vi "Task Manager.vi"() -> ()   [LabVIEW 2017]
doc: "Use this template to build a user interface event handler design pattern. Use this pattern for dialog boxes and other user interfaces. You also can create and execute user-defined events that the VI can handle the same way as user interface events."
uses:
  Task View Control.ctl
panel:
  in  "Advance":bool
  out "Input Task Tip":string
  in  "Input Value":string caption="Thermocouple Reading"
  out "Task Tip":string
  out "Experiment Progress":u8(slide) scale=0.0..15.0
  in  "?":bool
  out "tracker2":bool caption="Item 2"
  out "tracker5":bool caption="Item 5"
  out "tracker3":bool caption="Item 3"
  out "tracker1":bool caption="Item 1"
  out "tracker4":bool caption="Item 4"
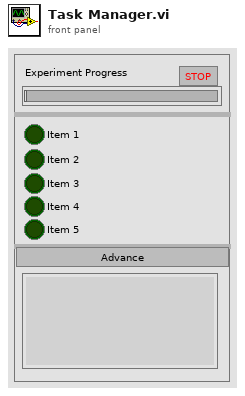
[diagram p1: front panel]
types:
  T1 = typedef "Task View Control.ctl" = enum16{"init", "Activate Pump 1", "Activate CTAH 1", "Set Pump Freq to 10Hz 1", "Vary Pump Freqs 1", "Vary Pump Freqs 2", "Stop Pump 1", "Stop Pump 2", "Ramp Up Pump Freq 1", "Ramp Up Pump Freq 2", "Ramp Up Pump Freq 3", "Ramp Up Pump Freq 4", "Ramp Up Power 1", "Ramp Up Power 2", "Ramp up Power 3", "Ramp up Power 4", "Ramp up Power 5", "Set CTAH 1", "Set CTAH 2", "Set CTAH 3", "Change Pump Freq", "Run Input 1", "Run Input 2", "Turn Off Power 1", "Turn Off Power 2", "Turn Off Power 3", "Primary Loop Cooldown 1", "Primary Loop Cooldown 2", "Primary Loop Cooldown 3", "Turn off CTAH", "Turn off chat", "complete"}
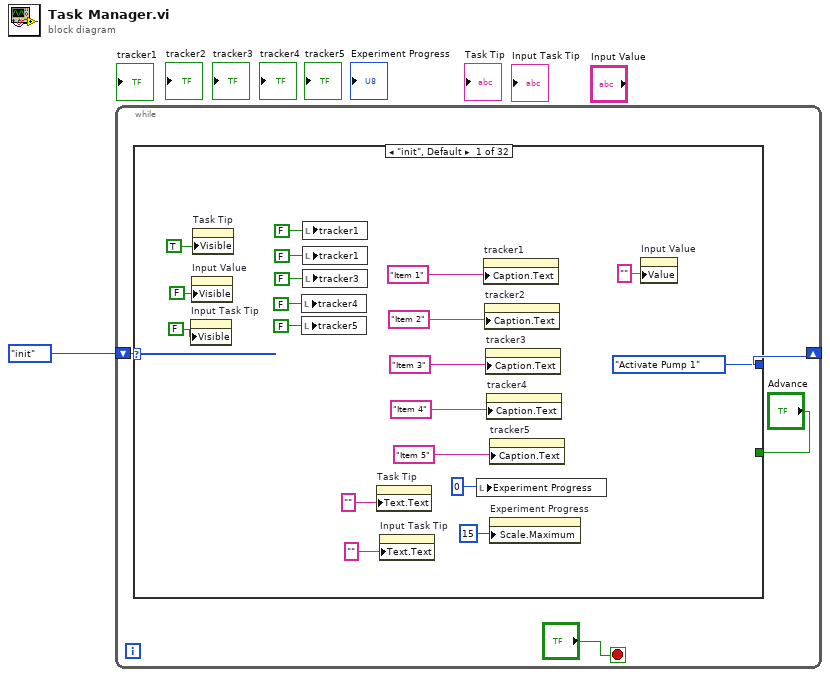
[diagram p0: block diagram]
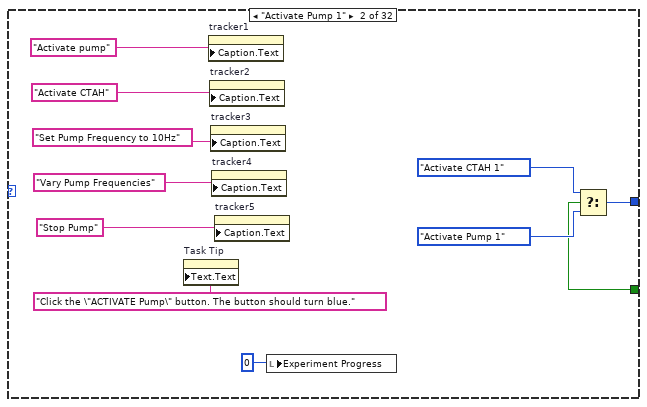
[diagram p2: hidden frame]
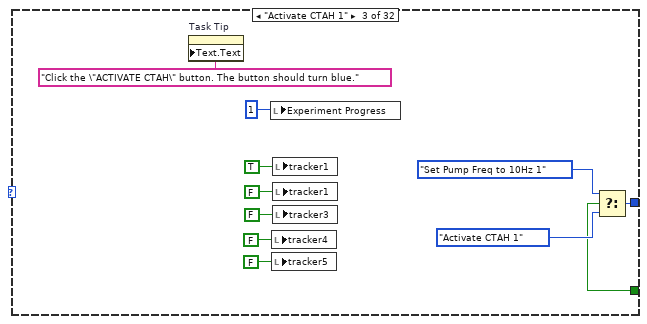
[diagram p3: hidden frame]
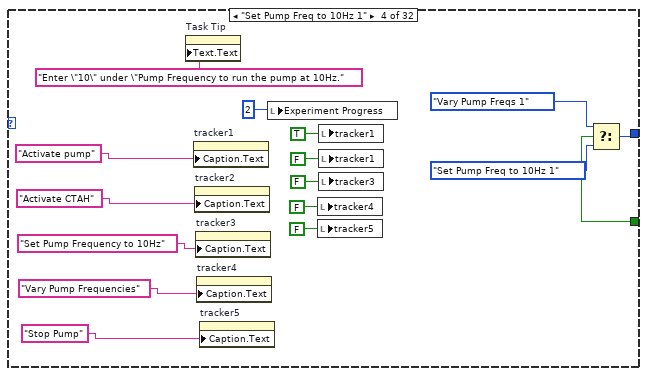
[diagram p4: hidden frame]
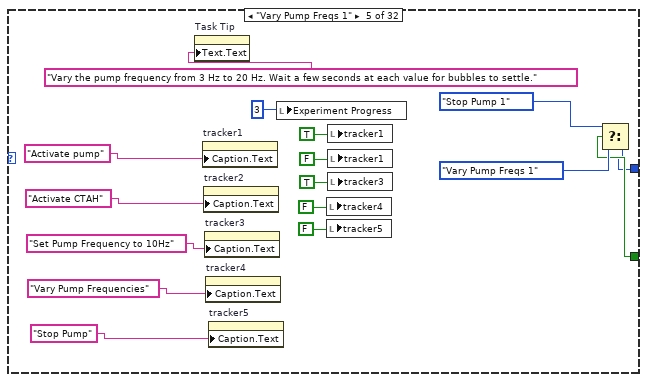
[diagram p5: hidden frame]
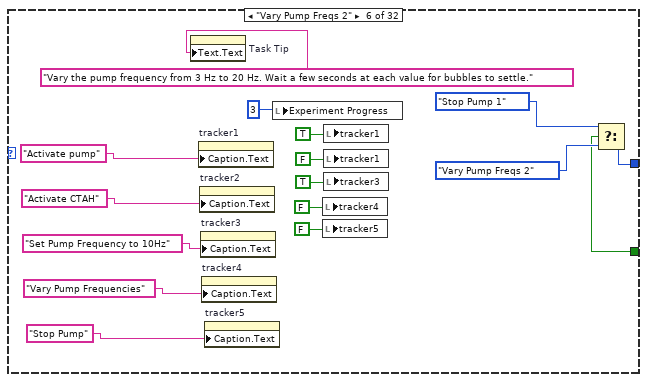
[diagram p6: hidden frame]
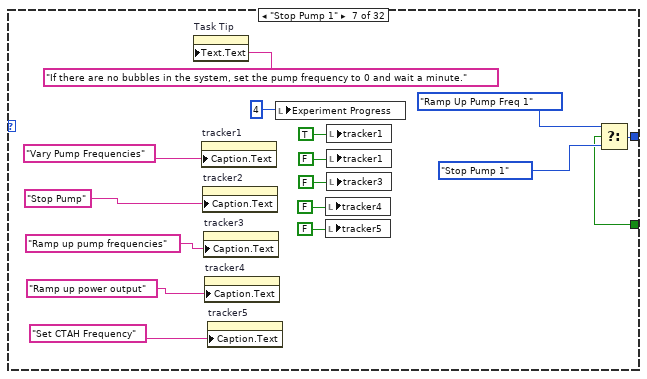
[diagram p7: hidden frame]
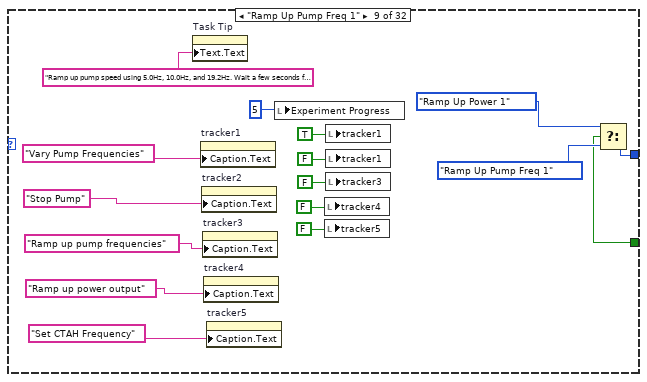
[diagram p9: hidden frame]
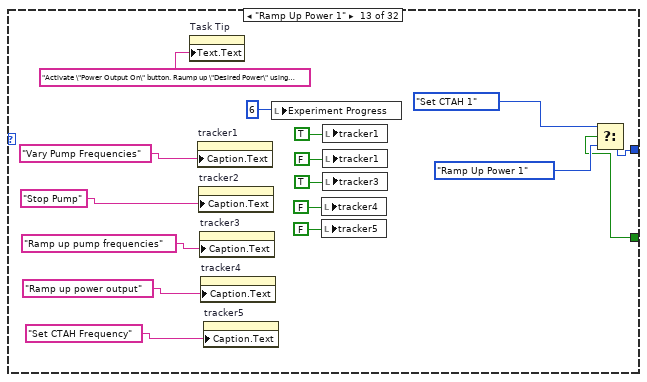
[diagram p13: hidden frame]
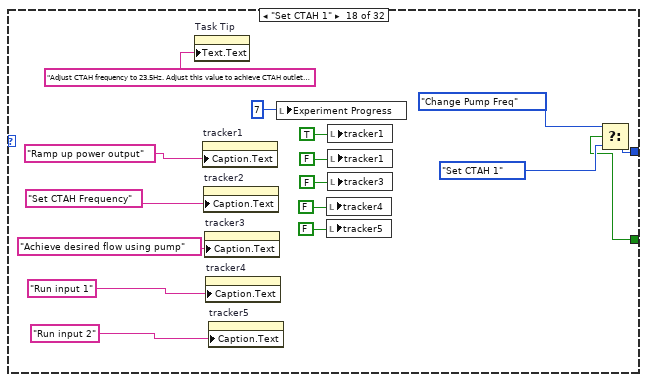
[diagram p18: hidden frame]
diagram:
  n1 = while {
    shift-right: [w3] -> _
    shift-left: Task_View_Control."init" -> [w4]
    stop <- "?" stop-if-true
    n2 = case shown="\"init\", Default" w4 {
      tunnel: [Task_View_Control."Activate Pump 1" w29 w45 w63 w66 w83 w100 _ w117 _ _ _ w134 _ _ _ _ w151 _ _ w168 w186 w202 w220 _ _ w236 _ _ w253 w270 w289] -> w3
      tunnel: "Advance" -> [_ w26 w43 w60 w67 w84 w101 _ w118 _ _ _ w135 _ _ _ _ w152 _ _ w169 w185 w203 w219 _ _ w237 _ _ w254 w271 w288]
      frame "init", Default {
        n3 = property on="Input Task Tip" class="Str"("Visible"=FALSE) -> ()  [unwired: 2 in, 2 out]
        n4 = property on="Input Value" class="Str"("Visible"=FALSE) -> ()  [unwired: 2 in, 2 out]
        n5 = property on="Task Tip" class="Str"("Visible"=TRUE) -> ()  [unwired: 2 in, 2 out]
        n6 = local write "tracker4"(FALSE) -> ()
        n7 = local write "tracker5"(FALSE) -> ()
        n8 = local write "tracker1"(FALSE) -> ()
        n9 = local write "tracker2"(FALSE) -> ()
        n10 = local write "tracker1"(FALSE) -> ()
        n11 = local write "tracker3"(FALSE) -> ()
        n12 = property on="Task Tip" class="Str"("Text.Text"="") -> ()  [unwired: 2 in, 2 out]
        n13 = property on="Input Task Tip" class="Str"("Text.Text"="") -> ()  [unwired: 2 in, 2 out]
        n14 = local write "Experiment Progress"(0) -> ()
        n15 = property on="tracker1" class="Bool (strict)"("Caption.Text"="Item 1") -> ()  [unwired: 2 in, 2 out]
        n16 = property on="tracker2" class="Bool (strict)"("Caption.Text"="Item 2") -> ()  [unwired: 2 in, 2 out]
        n17 = property on="tracker3" class="Bool (strict)"("Caption.Text"="Item 3") -> ()  [unwired: 2 in, 2 out]
        n18 = property on="tracker4" class="Bool (strict)"("Caption.Text"="Item 4") -> ()  [unwired: 2 in, 2 out]
        n19 = property on="tracker5" class="Bool (strict)"("Caption.Text"="Item 5") -> ()  [unwired: 2 in, 2 out]
        n20 = property on="Experiment Progress" class="Slide (strict)"("Scale.Maximum"=15) -> ()  [unwired: 2 in, 2 out]
        n21 = property on="Input Value" class="Str"("Value"="") -> ()  [unwired: 2 in, 2 out]
      }
      frame "Activate Pump 1" {
        n22 = property on="Task Tip" class="Str"("Text.Text"="Click the \"ACTIVATE Pump\" button. The button should turn blue.") -> ()  [unwired: 2 in, 2 out]
        n23 = property on="tracker1" class="Bool (strict)"("Caption.Text"="Activate pump") -> ()  [unwired: 2 in, 2 out]
        n24 = property on="tracker2" class="Bool (strict)"("Caption.Text"="Activate CTAH") -> ()  [unwired: 2 in, 2 out]
        n25 = property on="tracker3" class="Bool (strict)"("Caption.Text"="Set Pump Frequency to 10Hz") -> ()  [unwired: 2 in, 2 out]
        n26 = property on="tracker4" class="Bool (strict)"("Caption.Text"="Vary Pump Frequencies") -> ()  [unwired: 2 in, 2 out]
        n27 = property on="tracker5" class="Bool (strict)"("Caption.Text"="Stop Pump") -> ()  [unwired: 2 in, 2 out]
        n28 = local write "Experiment Progress"(0) -> ()
        n29 = Select(t=Task_View_Control."Activate CTAH 1", s=w26, f=Task_View_Control."Activate Pump 1") -> (s? t:f=w29:T1)
      }
      frame "Activate CTAH 1" {
        n30 = property on="Task Tip" class="Str"("Text.Text"="Click the \"ACTIVATE CTAH\" button. The button should turn blue.") -> ()  [unwired: 2 in, 2 out]
        n31 = local write "Experiment Progress"(1) -> ()
        n32 = local write "tracker4"(FALSE) -> ()
        n33 = local write "tracker5"(FALSE) -> ()
        n34 = local write "tracker1"(TRUE) -> ()
        n35 = local write "tracker2"(FALSE) -> ()
        n36 = local write "tracker1"(FALSE) -> ()
        n37 = local write "tracker3"(FALSE) -> ()
        n38 = Select(t=Task_View_Control."Set Pump Freq to 10Hz 1", s=w43, f=Task_View_Control."Activate CTAH 1") -> (s? t:f=w45:T1)
      }
      frame "Set Pump Freq to 10Hz 1" {
        n39 = property on="Task Tip" class="Str"("Text.Text"="Enter \"10\" under \"Pump Frequency to run the pump at 10Hz.") -> ()  [unwired: 2 in, 2 out]
        n40 = property on="tracker1" class="Bool (strict)"("Caption.Text"="Activate pump") -> ()  [unwired: 2 in, 2 out]
        n41 = property on="tracker2" class="Bool (strict)"("Caption.Text"="Activate CTAH") -> ()  [unwired: 2 in, 2 out]
        n42 = property on="tracker3" class="Bool (strict)"("Caption.Text"="Set Pump Frequency to 10Hz") -> ()  [unwired: 2 in, 2 out]
        n43 = property on="tracker4" class="Bool (strict)"("Caption.Text"="Vary Pump Frequencies") -> ()  [unwired: 2 in, 2 out]
        n44 = property on="tracker5" class="Bool (strict)"("Caption.Text"="Stop Pump") -> ()  [unwired: 2 in, 2 out]
        n45 = local write "Experiment Progress"(2) -> ()
        n46 = local write "tracker4"(FALSE) -> ()
        n47 = local write "tracker5"(FALSE) -> ()
        n48 = local write "tracker1"(TRUE) -> ()
        n49 = local write "tracker2"(TRUE) -> ()
        n50 = local write "tracker1"(FALSE) -> ()
        n51 = local write "tracker3"(FALSE) -> ()
        n52 = Select(t=Task_View_Control."Vary Pump Freqs 1", s=w60, f=Task_View_Control."Set Pump Freq to 10Hz 1") -> (s? t:f=w63:T1)
      }
      frame "Vary Pump Freqs 1" {
        n53 = property on="Task Tip" class="Str"("Text.Text"="Vary the pump frequency from 3 Hz to 20 Hz. Wait a few seconds at each value for bubbles to settle.") -> ()  [unwired: 2 in, 2 out]
        n54 = property on="tracker1" class="Bool (strict)"("Caption.Text"="Activate pump") -> ()  [unwired: 2 in, 2 out]
        n55 = property on="tracker2" class="Bool (strict)"("Caption.Text"="Activate CTAH") -> ()  [unwired: 2 in, 2 out]
        n56 = property on="tracker3" class="Bool (strict)"("Caption.Text"="Set Pump Frequency to 10Hz") -> ()  [unwired: 2 in, 2 out]
        n57 = property on="tracker4" class="Bool (strict)"("Caption.Text"="Vary Pump Frequencies") -> ()  [unwired: 2 in, 2 out]
        n58 = property on="tracker5" class="Bool (strict)"("Caption.Text"="Stop Pump") -> ()  [unwired: 2 in, 2 out]
        n59 = local write "Experiment Progress"(3) -> ()
        n60 = local write "tracker4"(FALSE) -> ()
        n61 = local write "tracker5"(FALSE) -> ()
        n62 = local write "tracker1"(TRUE) -> ()
        n63 = local write "tracker2"(TRUE) -> ()
        n64 = local write "tracker1"(FALSE) -> ()
        n65 = local write "tracker3"(TRUE) -> ()
        n66 = Select(t=Task_View_Control."Stop Pump 1", s=w67, f=Task_View_Control."Vary Pump Freqs 1") -> (s? t:f=w66:T1)
      }
      frame "Vary Pump Freqs 2" {
        n67 = property on="Task Tip" class="Str"("Text.Text"="Vary the pump frequency from 3 Hz to 20 Hz. Wait a few seconds at each value for bubbles to settle.") -> ()  [unwired: 2 in, 2 out]
        n68 = property on="tracker1" class="Bool (strict)"("Caption.Text"="Activate pump") -> ()  [unwired: 2 in, 2 out]
        n69 = property on="tracker2" class="Bool (strict)"("Caption.Text"="Activate CTAH") -> ()  [unwired: 2 in, 2 out]
        n70 = property on="tracker3" class="Bool (strict)"("Caption.Text"="Set Pump Frequency to 10Hz") -> ()  [unwired: 2 in, 2 out]
        n71 = property on="tracker4" class="Bool (strict)"("Caption.Text"="Vary Pump Frequencies") -> ()  [unwired: 2 in, 2 out]
        n72 = property on="tracker5" class="Bool (strict)"("Caption.Text"="Stop Pump") -> ()  [unwired: 2 in, 2 out]
        n73 = local write "Experiment Progress"(3) -> ()
        n74 = local write "tracker4"(FALSE) -> ()
        n75 = local write "tracker5"(FALSE) -> ()
        n76 = local write "tracker1"(TRUE) -> ()
        n77 = local write "tracker2"(TRUE) -> ()
        n78 = local write "tracker1"(FALSE) -> ()
        n79 = local write "tracker3"(TRUE) -> ()
        n80 = Select(t=Task_View_Control."Stop Pump 1", s=w84, f=Task_View_Control."Vary Pump Freqs 2") -> (s? t:f=w83:T1)
      }
      frame "Stop Pump 1" {
        n81 = property on="Task Tip" class="Str"("Text.Text"="If there are no bubbles in the system, set the pump frequency to 0 and wait a minute.") -> ()  [unwired: 2 in, 2 out]
        n82 = property on="tracker1" class="Bool (strict)"("Caption.Text"="Vary Pump Frequencies") -> ()  [unwired: 2 in, 2 out]
        n83 = property on="tracker2" class="Bool (strict)"("Caption.Text"="Stop Pump") -> ()  [unwired: 2 in, 2 out]
        n84 = property on="tracker3" class="Bool (strict)"("Caption.Text"="Ramp up pump frequencies") -> ()  [unwired: 2 in, 2 out]
        n85 = property on="tracker4" class="Bool (strict)"("Caption.Text"="Ramp up power output") -> ()  [unwired: 2 in, 2 out]
        n86 = property on="tracker5" class="Bool (strict)"("Caption.Text"="Set CTAH Frequency") -> ()  [unwired: 2 in, 2 out]
        n87 = local write "Experiment Progress"(4) -> ()
        n88 = local write "tracker4"(FALSE) -> ()
        n89 = local write "tracker5"(FALSE) -> ()
        n90 = local write "tracker1"(TRUE) -> ()
        n91 = local write "tracker2"(FALSE) -> ()
        n92 = local write "tracker1"(FALSE) -> ()
        n93 = local write "tracker3"(FALSE) -> ()
        n94 = Select(t=Task_View_Control."Ramp Up Pump Freq 1", s=w101, f=Task_View_Control."Stop Pump 1") -> (s? t:f=w100:T1)
      }
      frame "Stop Pump 2" {
      }
      frame "Ramp Up Pump Freq 1" {
        n95 = property on="Task Tip" class="Str"("Text.Text"="Ramp up pump speed using 5.0Hz, 10.0Hz, and 19.2Hz. Wait a few seconds for the system to settle at each value. Change the final value to achieve a mass flow of 0.18 kg/s.") -> ()  [unwired: 2 in, 2 out]
        n96 = property on="tracker1" class="Bool (strict)"("Caption.Text"="Vary Pump Frequencies") -> ()  [unwired: 2 in, 2 out]
        n97 = property on="tracker2" class="Bool (strict)"("Caption.Text"="Stop Pump") -> ()  [unwired: 2 in, 2 out]
        n98 = property on="tracker3" class="Bool (strict)"("Caption.Text"="Ramp up pump frequencies") -> ()  [unwired: 2 in, 2 out]
        n99 = property on="tracker4" class="Bool (strict)"("Caption.Text"="Ramp up power output") -> ()  [unwired: 2 in, 2 out]
        n100 = property on="tracker5" class="Bool (strict)"("Caption.Text"="Set CTAH Frequency") -> ()  [unwired: 2 in, 2 out]
        n101 = local write "Experiment Progress"(5) -> ()
        n102 = local write "tracker4"(FALSE) -> ()
        n103 = local write "tracker5"(FALSE) -> ()
        n104 = local write "tracker1"(TRUE) -> ()
        n105 = local write "tracker2"(TRUE) -> ()
        n106 = local write "tracker1"(FALSE) -> ()
        n107 = local write "tracker3"(FALSE) -> ()
        n108 = Select(t=Task_View_Control."Ramp Up Power 1", s=w118, f=Task_View_Control."Ramp Up Pump Freq 1") -> (s? t:f=w117:T1)
      }
      frame "Ramp Up Pump Freq 2" {
      }
      frame "Ramp Up Pump Freq 3" {
      }
      frame "Ramp Up Pump Freq 4" {
      }
      frame "Ramp Up Power 1" {
        n109 = property on="Task Tip" class="Str"("Text.Text"="Activate \"Power Output On\" button. Raump up \"Desired Power\" using 500W, 2000W, 4000W, 6000W, 8000W. Wait for 10 seconds at each value.") -> ()  [unwired: 2 in, 2 out]
        n110 = property on="tracker1" class="Bool (strict)"("Caption.Text"="Vary Pump Frequencies") -> ()  [unwired: 2 in, 2 out]
        n111 = property on="tracker2" class="Bool (strict)"("Caption.Text"="Stop Pump") -> ()  [unwired: 2 in, 2 out]
        n112 = property on="tracker3" class="Bool (strict)"("Caption.Text"="Ramp up pump frequencies") -> ()  [unwired: 2 in, 2 out]
        n113 = property on="tracker4" class="Bool (strict)"("Caption.Text"="Ramp up power output") -> ()  [unwired: 2 in, 2 out]
        n114 = property on="tracker5" class="Bool (strict)"("Caption.Text"="Set CTAH Frequency") -> ()  [unwired: 2 in, 2 out]
        n115 = local write "Experiment Progress"(6) -> ()
        n116 = local write "tracker4"(FALSE) -> ()
        n117 = local write "tracker5"(FALSE) -> ()
        n118 = local write "tracker1"(TRUE) -> ()
        n119 = local write "tracker2"(TRUE) -> ()
        n120 = local write "tracker1"(FALSE) -> ()
        n121 = local write "tracker3"(TRUE) -> ()
        n122 = Select(t=Task_View_Control."Set CTAH 1", s=w135, f=Task_View_Control."Ramp Up Power 1") -> (s? t:f=w134:T1)
      }
      frame "Ramp Up Power 2" {
      }
      frame "Ramp up Power 3" {
      }
      frame "Ramp up Power 4" {
      }
      frame "Ramp up Power 5" {
      }
      frame "Set CTAH 1" {
        n123 = property on="Task Tip" class="Str"("Text.Text"="Adjust CTAH frequency to 23.5Hz. Adjust this value to achieve CTAH outlet temperature of 80°C.") -> ()  [unwired: 2 in, 2 out]
        n124 = property on="tracker1" class="Bool (strict)"("Caption.Text"="Ramp up power output") -> ()  [unwired: 2 in, 2 out]
        n125 = property on="tracker2" class="Bool (strict)"("Caption.Text"="Set CTAH Frequency") -> ()  [unwired: 2 in, 2 out]
        n126 = property on="tracker3" class="Bool (strict)"("Caption.Text"="Achieve desired flow using pump") -> ()  [unwired: 2 in, 2 out]
        n127 = property on="tracker4" class="Bool (strict)"("Caption.Text"="Run input 1") -> ()  [unwired: 2 in, 2 out]
        n128 = property on="tracker5" class="Bool (strict)"("Caption.Text"="Run input 2") -> ()  [unwired: 2 in, 2 out]
        n129 = local write "Experiment Progress"(7) -> ()
        n130 = local write "tracker4"(FALSE) -> ()
        n131 = local write "tracker5"(FALSE) -> ()
        n132 = local write "tracker1"(TRUE) -> ()
        n133 = local write "tracker2"(FALSE) -> ()
        n134 = local write "tracker1"(FALSE) -> ()
        n135 = local write "tracker3"(FALSE) -> ()
        n136 = Select(t=Task_View_Control."Change Pump Freq", s=w152, f=Task_View_Control."Set CTAH 1") -> (s? t:f=w151:T1)
      }
      frame "Set CTAH 2" {
      }
      frame "Set CTAH 3" {
      }
      frame "Change Pump Freq" {
        n137 = property on="Task Tip" class="Str"("Text.Text"="Adjust pump frequency to achieve mass flow rate of 0.18 kg/s.") -> ()  [unwired: 2 in, 2 out]
        n138 = property on="tracker1" class="Bool (strict)"("Caption.Text"="Ramp up power output") -> ()  [unwired: 2 in, 2 out]
        n139 = property on="tracker2" class="Bool (strict)"("Caption.Text"="Set CTAH Frequency") -> ()  [unwired: 2 in, 2 out]
        n140 = property on="tracker3" class="Bool (strict)"("Caption.Text"="Achieve desired flow using pump") -> ()  [unwired: 2 in, 2 out]
        n141 = property on="tracker4" class="Bool (strict)"("Caption.Text"="Run input 1") -> ()  [unwired: 2 in, 2 out]
        n142 = property on="tracker5" class="Bool (strict)"("Caption.Text"="Run input 2") -> ()  [unwired: 2 in, 2 out]
        n143 = local write "Experiment Progress"(8) -> ()
        n144 = local write "tracker4"(FALSE) -> ()
        n145 = local write "tracker5"(FALSE) -> ()
        n146 = local write "tracker1"(TRUE) -> ()
        n147 = local write "tracker2"(TRUE) -> ()
        n148 = local write "tracker1"(FALSE) -> ()
        n149 = local write "tracker3"(FALSE) -> ()
        n150 = Select(t=Task_View_Control."Run Input 1", s=w169, f=Task_View_Control."Change Pump Freq") -> (s? t:f=w168:T1)
      }
      frame "Run Input 1" {
        n151 = property on="Task Tip" class="Str"("Text.Text"="Run input 1. This will take a while.") -> ()  [unwired: 2 in, 2 out]
        n152 = property on="tracker1" class="Bool (strict)"("Caption.Text"="Ramp up power output") -> ()  [unwired: 2 in, 2 out]
        n153 = property on="tracker2" class="Bool (strict)"("Caption.Text"="Set CTAH Frequency") -> ()  [unwired: 2 in, 2 out]
        n154 = property on="tracker3" class="Bool (strict)"("Caption.Text"="Achieve desired flow using pump") -> ()  [unwired: 2 in, 2 out]
        n155 = property on="tracker4" class="Bool (strict)"("Caption.Text"="Run input 1") -> ()  [unwired: 2 in, 2 out]
        n156 = property on="tracker5" class="Bool (strict)"("Caption.Text"="Run input 2") -> ()  [unwired: 2 in, 2 out]
        n157 = local write "Experiment Progress"(9) -> ()
        n158 = local write "tracker4"(FALSE) -> ()
        n159 = local write "tracker5"(FALSE) -> ()
        n160 = local write "tracker1"(TRUE) -> ()
        n161 = local write "tracker2"(TRUE) -> ()
        n162 = local write "tracker1"(FALSE) -> ()
        n163 = local write "tracker3"(TRUE) -> ()
        n164 = Select(t=Task_View_Control."Run Input 2", s=w185, f=Task_View_Control."Run Input 1") -> (s? t:f=w186:T1)
      }
      frame "Run Input 2" {
        n165 = property on="Task Tip" class="Str"("Text.Text"="Run input 2. This will take a while.") -> ()  [unwired: 2 in, 2 out]
        n166 = property on="tracker1" class="Bool (strict)"("Caption.Text"="Run input 1") -> ()  [unwired: 2 in, 2 out]
        n167 = property on="tracker2" class="Bool (strict)"("Caption.Text"="Run input 2") -> ()  [unwired: 2 in, 2 out]
        n168 = property on="tracker3" class="Bool (strict)"("Caption.Text"="Turn off power") -> ()  [unwired: 2 in, 2 out]
        n169 = property on="tracker4" class="Bool (strict)"("Caption.Text"="Primary loop cooldown") -> ()  [unwired: 2 in, 2 out]
        n170 = property on="tracker5" class="Bool (strict)"("Caption.Text"="Turn off CTAH") -> ()  [unwired: 2 in, 2 out]
        n171 = local write "Experiment Progress"(10) -> ()
        n172 = local write "tracker4"(FALSE) -> ()
        n173 = local write "tracker5"(FALSE) -> ()
        n174 = local write "tracker1"(TRUE) -> ()
        n175 = local write "tracker2"(FALSE) -> ()
        n176 = local write "tracker1"(FALSE) -> ()
        n177 = local write "tracker3"(FALSE) -> ()
        n178 = Select(t=Task_View_Control."Turn Off Power 1", s=w203, f=Task_View_Control."Run Input 2") -> (s? t:f=w202:T1)
      }
      frame "Turn Off Power 1" {
        n179 = property on="Task Tip" class="Str"("Text.Text"="Set \"Desired Power\" to 0W. Once the output power value is at 0W, click the \"Power Output On\" button. It should turn grey to indicate it is off.") -> ()  [unwired: 2 in, 2 out]
        n180 = property on="tracker1" class="Bool (strict)"("Caption.Text"="Run input 1") -> ()  [unwired: 2 in, 2 out]
        n181 = property on="tracker2" class="Bool (strict)"("Caption.Text"="Run input 2") -> ()  [unwired: 2 in, 2 out]
        n182 = property on="tracker3" class="Bool (strict)"("Caption.Text"="Turn off power") -> ()  [unwired: 2 in, 2 out]
        n183 = property on="tracker4" class="Bool (strict)"("Caption.Text"="Primary loop cooldown") -> ()  [unwired: 2 in, 2 out]
        n184 = property on="tracker5" class="Bool (strict)"("Caption.Text"="Turn off CTAH and Pump") -> ()  [unwired: 2 in, 2 out]
        n185 = local write "Experiment Progress"(11) -> ()
        n186 = local write "tracker4"(FALSE) -> ()
        n187 = local write "tracker5"(FALSE) -> ()
        n188 = local write "tracker1"(TRUE) -> ()
        n189 = local write "tracker2"(TRUE) -> ()
        n190 = local write "tracker1"(FALSE) -> ()
        n191 = local write "tracker3"(FALSE) -> ()
        n192 = Select(t=Task_View_Control."Primary Loop Cooldown 1", s=w219, f=Task_View_Control."Turn Off Power 1") -> (s? t:f=w220:T1)
      }
      frame "Turn Off Power 2" {
      }
      frame "Turn Off Power 3" {
      }
      frame "Primary Loop Cooldown 1" {
        n193 = property on="Task Tip" class="Str"("Text.Text"="Set CTAH frequency to 60. Once the bulk temperature fluids decrease below 40°C, stop the CTAH by setting its frequency to 0Hz.") -> ()  [unwired: 2 in, 2 out]
        n194 = property on="tracker1" class="Bool (strict)"("Caption.Text"="Run input 1") -> ()  [unwired: 2 in, 2 out]
        n195 = property on="tracker2" class="Bool (strict)"("Caption.Text"="Turn off power") -> ()  [unwired: 2 in, 2 out]
        n196 = property on="tracker3" class="Bool (strict)"("Caption.Text"="Primary loop cooldown") -> ()  [unwired: 2 in, 2 out]
        n197 = property on="tracker4" class="Bool (strict)"("Caption.Text"="Turn off CTAH and Pump") -> ()  [unwired: 2 in, 2 out]
        n198 = property on="tracker5" class="Bool (strict)"("Caption.Text"="Turn off chat") -> ()  [unwired: 2 in, 2 out]
        n199 = local write "Experiment Progress"(12) -> ()
        n200 = local write "tracker4"(FALSE) -> ()
        n201 = local write "tracker5"(FALSE) -> ()
        n202 = local write "tracker1"(TRUE) -> ()
        n203 = local write "tracker2"(TRUE) -> ()
        n204 = local write "tracker1"(FALSE) -> ()
        n205 = local write "tracker3"(FALSE) -> ()
        n206 = Select(t=Task_View_Control."Turn off CTAH", s=w237, f=Task_View_Control."Primary Loop Cooldown 1") -> (s? t:f=w236:T1)
      }
      frame "Primary Loop Cooldown 2" {
      }
      frame "Primary Loop Cooldown 3" {
      }
      frame "Turn off CTAH" {
        n207 = property on="Task Tip" class="Str"("Text.Text"="Press the \"ACTIVATE CTAH\" button to turn off CTAH control. Set the pump frequency to 0Hz and press the \"ACTIVATE Pump\" button to shut it off.") -> ()  [unwired: 2 in, 2 out]
        n208 = property on="tracker1" class="Bool (strict)"("Caption.Text"="Run input 1") -> ()  [unwired: 2 in, 2 out]
        n209 = property on="tracker2" class="Bool (strict)"("Caption.Text"="Turn off power") -> ()  [unwired: 2 in, 2 out]
        n210 = property on="tracker3" class="Bool (strict)"("Caption.Text"="Primary loop cooldown") -> ()  [unwired: 2 in, 2 out]
        n211 = property on="tracker4" class="Bool (strict)"("Caption.Text"="Turn off CTAH and Pump") -> ()  [unwired: 2 in, 2 out]
        n212 = property on="tracker5" class="Bool (strict)"("Caption.Text"="Turn off chat") -> ()  [unwired: 2 in, 2 out]
        n213 = local write "Experiment Progress"(13) -> ()
        n214 = local write "tracker4"(FALSE) -> ()
        n215 = local write "tracker5"(FALSE) -> ()
        n216 = local write "tracker1"(TRUE) -> ()
        n217 = local write "tracker2"(TRUE) -> ()
        n218 = local write "tracker1"(FALSE) -> ()
        n219 = local write "tracker3"(TRUE) -> ()
        n220 = Select(t=Task_View_Control."Turn off chat", s=w254, f=Task_View_Control."Turn off CTAH") -> (s? t:f=w253:T1)
      }
      frame "Turn off chat" {
        n221 = property on="Task Tip" class="Str"("Text.Text"="Look at the chat window. Click \"Stop Reading\", \"Save Log\" and then \"Stop Chat.\"") -> ()  [unwired: 2 in, 2 out]
        n222 = property on="tracker1" class="Bool (strict)"("Caption.Text"="Run input 1") -> ()  [unwired: 2 in, 2 out]
        n223 = property on="tracker2" class="Bool (strict)"("Caption.Text"="Turn off power") -> ()  [unwired: 2 in, 2 out]
        n224 = property on="tracker3" class="Bool (strict)"("Caption.Text"="Primary loop cooldown") -> ()  [unwired: 2 in, 2 out]
        n225 = property on="tracker4" class="Bool (strict)"("Caption.Text"="Turn off CTAH and Pump") -> ()  [unwired: 2 in, 2 out]
        n226 = property on="tracker5" class="Bool (strict)"("Caption.Text"="Turn off chat") -> ()  [unwired: 2 in, 2 out]
        n227 = local write "Experiment Progress"(14) -> ()
        n228 = local write "tracker4"(TRUE) -> ()
        n229 = local write "tracker5"(FALSE) -> ()
        n230 = local write "tracker1"(TRUE) -> ()
        n231 = local write "tracker2"(TRUE) -> ()
        n232 = local write "tracker1"(FALSE) -> ()
        n233 = local write "tracker3"(TRUE) -> ()
        n234 = Select(t=Task_View_Control."complete", s=w271, f=Task_View_Control."Turn off chat") -> (s? t:f=w270:T1)
      }
      frame "complete" {
        n235 = property on="Task Tip" class="Str"("Text.Text"="Experiment complete. Press \"STOP\" at the top of this window.") -> ()  [unwired: 2 in, 2 out]
        n236 = property on="tracker1" class="Bool (strict)"("Caption.Text"="Run input 1") -> ()  [unwired: 2 in, 2 out]
        n237 = property on="tracker2" class="Bool (strict)"("Caption.Text"="Turn off power") -> ()  [unwired: 2 in, 2 out]
        n238 = property on="tracker3" class="Bool (strict)"("Caption.Text"="Primary loop cooldown") -> ()  [unwired: 2 in, 2 out]
        n239 = property on="tracker4" class="Bool (strict)"("Caption.Text"="Turn off CTAH and Pump") -> ()  [unwired: 2 in, 2 out]
        n240 = property on="tracker5" class="Bool (strict)"("Caption.Text"="Turn off chat") -> ()  [unwired: 2 in, 2 out]
        n241 = local write "Experiment Progress"(15) -> ()
        n242 = local write "tracker2"(TRUE) -> ()
        n243 = local write "tracker1"(FALSE) -> ()
        n244 = local write "tracker3"(TRUE) -> ()
        n245 = local write "tracker4"(TRUE) -> ()
        n246 = local write "tracker5"(TRUE) -> ()
        n247 = property on="tracker1" class="Bool (strict)"("Value"=TRUE) -> ()  [unwired: 2 in, 2 out]
        n248 = Select(t=Task_View_Control."complete", s=w288, f=Task_View_Control."complete") -> (s? t:f=w289:T1)
      }
    }
  }
